vi "Initialize.vi"(8 "error in (no error)":errorcluster, 9 "Reset (True)":bool=TRUE, 10 "ID Query (True)":bool=TRUE, 11 "VISA resource name":refnum<visa-resource-name>) -> (0 "error out":errorcluster, 3 "VISA resource name out":refnum<visa-resource-name>)   [LabVIEW 2017, in "ADCMT 6240.lvlib"]
doc: "Establishes communication with the instrument and optionally performs an instrument identification query and/or an instrument reset. It also places the instrument in a default state needed for other instrument driver operations. Therefore, call this VI before calling other instrument driver VIs for this instrument. Generally, you need to call the Initialize VI only once at the beginning of an application."
uses:
  ADCMT 6240.lvlib
  Private/Extended User Data.ctl
panel:
  # "(c) 2008 ADC Corporation  ALL RIGHTS RESERVED."
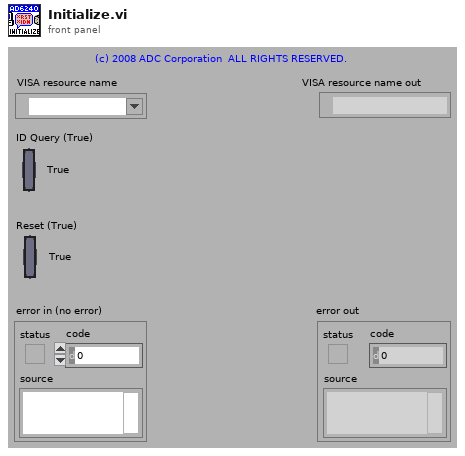
[diagram p1: front panel]
types:
  T1 = typedef "ADCMT 6240.lvlib/Extended User Data.ctl" = cluster{"Trigger Mode":u16, "Output Mode":u16, "Sample Count":i32, "Model":u16}
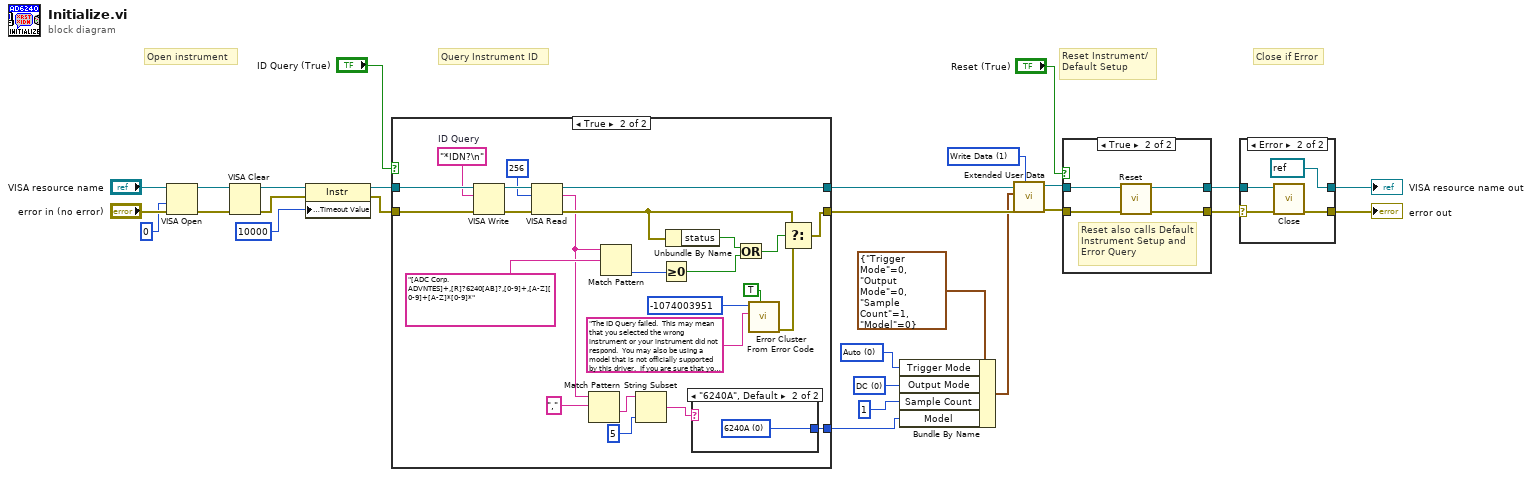
[diagram p0: block diagram]
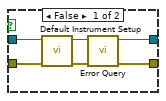
[diagram p3: hidden frame]
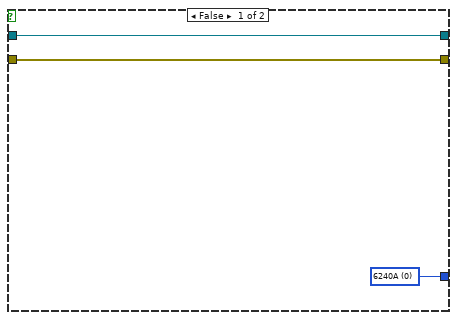
[diagram p4: hidden frame]
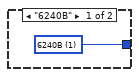
[diagram p5: hidden frame]
diagram:
  w3 = u16 0 items=["DC", "Pulse", "Sweep", "Pulse-Sweep"] ("Output Mode")
  w4 = u16 1 items=["Read Data", "Write Data", "Dispose of Data"] ("Action")
  w8 = u16 0 items=["Auto", "Manual"]
  # "Close if Error"
  # "Query Instrument ID"
  # "Reset Instrument/\nDefault Setup"
  # "Open instrument"
  n1 = VISA Open ("VISAオープン")(access mode=u32 0, error in (no error)="error in (no error)", VISA resource name="VISA resource name") -> (VISA resource name=w19:refnum<visa-resource-name>, error out=w18:errorcluster)  [unwired: 2 in]
  n2 = VISA Clear ("VISAクリア")(VISA resource name=w19, error in (no error)=w18) -> (VISA resource name out=w17:refnum<visa-resource-name>, error out=w16:errorcluster)
  n3 = property on="プロパティノード" class="Instr"(reference=w17, error in=w16, "General Settings:Timeout Value"=u32 10000) -> (reference out=w22:refnum<visa-resource-name>, error out=w21:errorcluster)
  n4 = case "ケースストラクチャ" shown="True" "ID Query (True)" {
    tunnel: [w29 w54] -> w7
    tunnel: [w30 w51] -> w6
    tunnel: w22 -> [w30 w52]
    tunnel: w21 -> [w29 w53]
    tunnel: [w28 w31] -> w1
    frame False {
      w28 = u16 0 items=["6240A", "6240B"] ("Model")
    }
    frame True {
      w37 = "*IDN?\n"  # ID Query
      n5 = VISA Write ("VISA書き込み")(VISA resource name=w52, write buffer=w37, error in (no error)=w53) -> (VISA resource name out=w50:refnum<visa-resource-name>, error out=w49:errorcluster)  [unwired: 1 out]
      n6 = VISA Read ("VISA読み取り")(VISA resource name=w50, byte count=u32 256, error in (no error)=w49) -> (VISA resource name out=w51:refnum<visa-resource-name>, read buffer=w33:string, error out=w41:errorcluster)  [unwired: 1 out]
      n7 = Match Pattern(string=w33, regular expression=",") -> (after substring=w35:string)  [unwired: 1 in, 3 out]
      n8 = Match Pattern ("パターンで一致")(string=w33, regular expression="[ADC Corp.ADVNTES]+,[R]?6240[AB]?,[0-9]+,[A-Z][0-9]+[A-Z]*[0-9]*") -> (offset past match=w42:i32)  [unwired: 1 in, 3 out]
      n9 = String Subset(string=w35, length (rest)=5 ("length (rest)")) -> (substring=w32:string)  [unwired: 1 in]
      n10 = Greater Or Equal To 0? ("0以上?")(x=w42) -> (x >= 0?=w39:bool)
      n11 = Unbundle By Name ("名前でバンドル解除")(w41) -> ("status"=w40:bool)
      n12 = case shown="\"6240A\", Default" w32 {
        tunnel: [w55 w56] -> w31
        frame "6240B" {
          w55 = u16 1 items=["6240A", "6240B"] ("Model")
        }
        frame "6240A", Default {
          w56 = u16 0 items=["6240A", "6240B"] ("Model")
        }
      }
      n13 = Or(x=w40, y=w39) -> (x .or. y?=w38:bool)
      n14 = call <vilib>:"Error Cluster From Error Code.vi"("show call chain? (False)"=TRUE, "error message (\"\")"="The ID Query failed.  This may mean that you selected the wrong instrument or your instrument did not respond.  You may also be using a model that is not officially supported by this driver.  If you are sure that you have selected the correct instrument and it is responding, try disabling the ID Query." ("Source (VI Name)"), "error code (0)"=-1074003951 ("Code")) -> ("error out"=w46:errorcluster)  [unwired: 6 in]
      n15 = Select ("選択")(t=w41, s=w38, f=w46) -> (s? t:f=w54:errorcluster)
    }
  }
  n16 = Bundle By Name ("名前でバンドル")(cluster=T1 {"Trigger Mode"=0, "Output Mode"=0, "Sample Count"=1, "Model"=0} ("User Data Definition"), "Trigger Mode"=w8, "Output Mode"=w3, "Sample Count"=1, "Model"=w1) -> (w5:T1)
  n17 = call "Extended User Data.vi"("Action"=w4, "Error In (no error)"=w7, "User Data In"=w5, "VISA resource name in"=w6) -> ("Error Out"=w10:errorcluster, "VISA resource name out"=w11:refnum<visa-resource-name>)  [unwired: 5 in, 1 out]
  n18 = case "ケースストラクチャ" shown="True" "Reset (True)" {
    tunnel: w10 -> [w61 w63]
    tunnel: [w58 w66] -> w12
    tunnel: w11 -> [w62 w64]
    tunnel: [w59 w65] -> w13
    frame False {
      n19 = call "Default Instrument Setup.vi"("error in (no error)"=w61, "VISA resource name"=w62) -> ("error out"=w57:errorcluster, "VISA resource name out"=w60:refnum<visa-resource-name>)  [unwired: 8 in]
      n20 = call "Error Query.vi"("error in (no error)"=w57, "VISA resource name"=w60) -> ("error out"=w58:errorcluster, "VISA resource name out"=w59:refnum<visa-resource-name>)  [unwired: 6 in, 2 out]
    }
    frame True {
      # "Reset also calls Default Instrument Setup and Error Query"
      n21 = call "Reset.vi"("error in (no error)"=w63, "VISA resource name"=w64) -> ("error out"=w66:errorcluster, "VISA resource name out"=w65:refnum<visa-resource-name>)  [unwired: 8 in]
    }
  }
  n22 = case "ケースストラクチャ" shown="Error" w12 {
    selector: w12 -> [w67 w70]
    tunnel: w13 -> [w68 w71]
    tunnel: [w68 refnum<visa-resource-name> refnum ("VISA resource name out")] -> w15
    tunnel: [w67 w72] -> w14
    frame No Error {
    }
    frame Error {
      n23 = call "Close.vi"("error in (no error)"=w70, "VISA resource name"=w71) -> ("error out"=w72:errorcluster)  [unwired: 9 in]
    }
  }
  "VISA resource name out" <- w15
  "error out" <- w14
